vi "Read Calibration Routine.vi"(8 "error in":errorcluster, 11 "Calibration Actor in":refnum<class "Calibration Actor.lvclass">) -> (0 "error out":errorcluster, 1 "Vals":string[](array[string]), 2 "tags":string[](array[string]), 3 "Calibration Actor out":refnum<class "Calibration Actor.lvclass">)   [LabVIEW 2018, in "Calibration.lvlib" / "Calibration Actor.lvclass"]
doc: "Parse the calibration file that is loaded and load the steps as necessary."
uses:
  Calibration Actor.lvclass
  <vilib>/regexp/Match Regular Expression.xnode
  Common/Wait/Wait STEP.lvclass
  Common/O2 Valve/O2 Valve STEP.lvclass
  reusable/Sequence/STEPS/STEP.lvclass
  Common/O2 Flow Rate/O2 Flow Rate STEP.lvclass
  Common/Speaker/Speaker STEP.lvclass
  Common/Filter/Filter Step/Filter STEP.lvclass
  Common/O3 Level/O3 Lamp Frequency STEP.lvclass
  Common/O3 Generator Power/O3 Generator Power STEP.lvclass
  reusable/Sequence/SEQ/SEQ.lvclass
  <vilib>/ActorFramework/Actor/Actor.lvclass
  Common/Set cycle state/Set cycle state STEP.lvclass
  Common/Denuder/Denuder STEP.lvclass
  reusable/Session APIs/CVT/CVT.lvclass
  Common/Reset Cycle State STEP/Reset cycle state STEP.lvclass
  Common/O3 Dump Rate Step/O3 Dump Rate STEP/O3 DumpRate STEP.lvclass
  Common/Pressure Control Rate STEP/Pressure Control Rate STEP.lvclass
  Common/Inlet STEP/Inlet STEP.lvclass
  <vilib>/ActorFramework/Message Enqueuer/Message Enqueuer.lvclass
  C:/Users/Labview/Documents/exscalabar_server/reusable/Sequence/STEPS/LEAVES/Switch/Switch Step.lvclass
  C:/Users/Labview/Documents/exscalabar_server/reusable/Sequence/STEPS/STEP.lvclass
  C:/Users/Labview/Documents/exscalabar_server/reusable/Sequence/STEPS/LEAVES/Double/Switch DBL.lvclass
  C:/Users/Labview/Documents/exscalabar_server/SuperActor/SuperActor.lvclass
  C:/Program Files (x86)/National Instruments/LabVIEW 2018/vi.lib/ActorFramework/Actor/Actor.lvclass
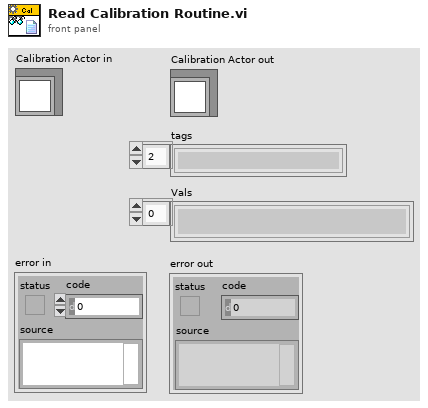
[diagram p1: front panel]
types:
  T1 = cluster{"Cycle":bool, "Period":i16, "Length":i16}
  T2 = typedef "Session - Root.lvclass/Session Handle.ctl" = refnum<data-value>
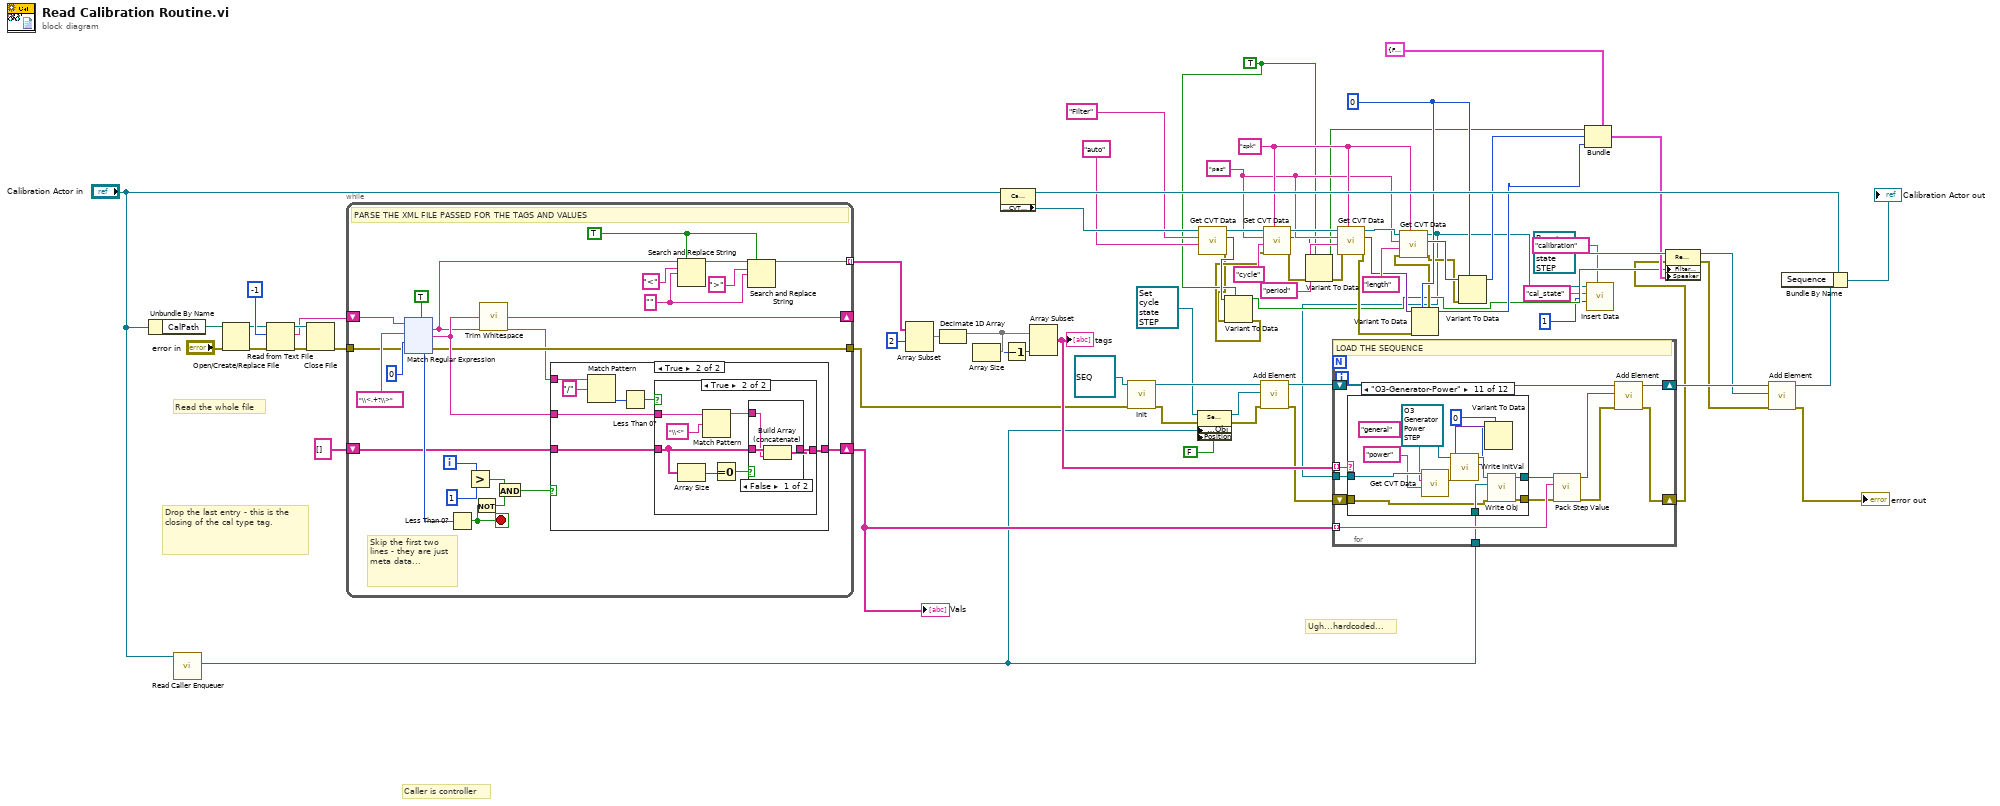
[diagram p0: block diagram]
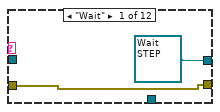
[diagram p2: hidden frame]
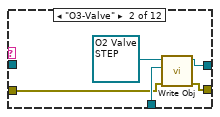
[diagram p3: hidden frame]
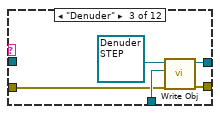
[diagram p4: hidden frame]
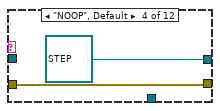
[diagram p5: hidden frame]
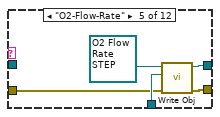
[diagram p6: hidden frame]
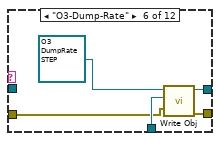
[diagram p7: hidden frame]
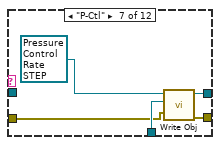
[diagram p8: hidden frame]
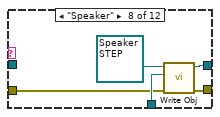
[diagram p9: hidden frame]
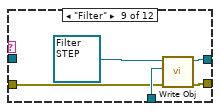
[diagram p10: hidden frame]
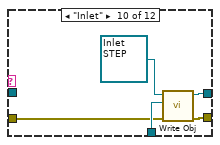
[diagram p11: hidden frame]
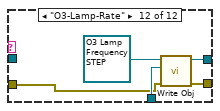
[diagram p12: hidden frame]
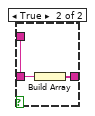
[diagram p15: hidden frame]
diagram:
  w22 = i16 0
  w27 = TRUE
  w33 = "pas" ("Group")
  w34 = "spk" ("Subgroup")
  # "Caller is controller"
  # "Ugh...hardcoded..."
  # "Read the whole file"
  # "Drop the last entry - this is the closing of the cal type tag."
  n1 = Unbundle By Name("Calibration Actor in") -> ("CalPath"=w44:path)
  n2 = call <vilib>:"Read Caller Enqueuer.vi"("Actor"="Calibration Actor in") -> ("Caller Enqueuer"=w50:refnum<class "Message Enqueuer.lvclass">)  [unwired: 10 in]
  n3 = Open/Create/Replace File(file path (use dialog)=w44, error in="error in") -> (refnum out=w71:refnum<file>, error out=w70:errorcluster)  [unwired: 4 in, 1 out]
  n4 = Read from Text File(file (use dialog)=w71, count=-1, error in=w70) -> (refnum out=w69:refnum<file>, text=w68:string, error out=w61:errorcluster)  [unwired: 1 in, 1 out]
  n5 = Close File(refnum=w69, error in=w61) -> (error out=w60:errorcluster)  [unwired: 1 out]
  n6 = while {
    shift-right: [w96] -> _
    shift-left: w68 -> [w95]
    shift-right: [w85] -> w55
    shift-left: string[] [] -> [w86]
    tunnel: w60 -> [w82]
    tunnel: [w81] -> w48
    tunnel: [w77] -> w59 mode=indexing
    i -> [w90]
    stop <- w83 stop-if-true
    w74 = "" ("replace string (\"\")")
    w76 = TRUE ("ignore case? (F)")
    # "Skip the first two lines - they are just meta data..."
    # "PARSE THE XML FILE PASSED FOR THE TAGS AND VALUES"
    n7 = xnode "Match Regular Expression"("input string"=w95, "regular expression"="\\<.+?\\>", "offset (0)"=0, "error in"=w82, "multiline? (F)"=TRUE) -> ("whole match"=w80:string, "after match"=w92:string, "offset past match"=w93:i32, "error out"=w81:errorcluster)  [unwired: 1 in, 1 out]
    n8 = Less Than 0?(x=w93) -> (x < 0?=w83:bool)
    n9 = Greater?(x=w90, y=1) -> (0:w88:bool)
    n10 = Not(x=w83) -> (.not. x?=w84:bool)
    n11 = call <vilib>:"Trim Whitespace.vi"("string"=w92) -> ("trimmed string"=w96:string)  [unwired: 1 in]
    n12 = And(x=w88, y=w84) -> (x .and. y?=w87:bool)
    n13 = case shown="True" w87 {
      tunnel: w80 -> [_ w105]
      tunnel: w92 -> [_ w101]
      tunnel: w86 -> [w98 w100]
      tunnel: [w98 w99] -> w85
      frame False {
      }
      frame True {
        n14 = Match Pattern(string=w105, regular expression="/") -> (offset past match=w103:i32)  [unwired: 1 in, 3 out]
        n15 = Less Than 0?(x=w103) -> (x < 0?=w102:bool)
        n16 = case shown="True" w102 {
          tunnel: w101 -> [_ w113]
          tunnel: w100 -> [w106 w108]
          tunnel: [w106 w109] -> w99
          frame False {
          }
          frame True {
            n17 = Array Size(array=w108) -> (size(s)=w110:i32)
            n18 = Match Pattern(string=w113, regular expression="\\<") -> (before substring=w107:string)  [unwired: 1 in, 3 out]
            n19 = Equal To 0?(x=w110) -> (x = 0?=w111:bool)
            n20 = case shown="False" w111 {
              tunnel: w107 -> [w114 w118]
              tunnel: [w115 w117] -> w109
              tunnel: w108 -> [w116 _]
              frame False {
                n21 = Build Array (concatenate)(w116, w114) -> (w115:string[])
              }
              frame True {
                n22 = Build Array(w118) -> (w117:string[])
              }
            }
          }
        }
      }
    }
    n23 = Search and Replace String(replace all?=w76, input string=w80, search string="<", replace string=w74) -> (result string=w78:string)  [unwired: 4 in, 3 out]
    n24 = Search and Replace String(replace all?=w76, input string=w78, search string=">", replace string=w74) -> (result string=w77:string)  [unwired: 4 in, 3 out]
  }
  "Vals" <- w55
  n25 = Array Subset(array=w59, index=2) -> (w65:string[])  [unwired: 1 in]
  n26 = Decimate 1D Array(w65) -> (w64:string[])  [unwired: 1 out]
  n27 = Array Size(array=w64) -> (size(s)=w63:i32)
  n28 = property class="Calibration Actor"(reference="Calibration Actor in") -> (reference out=w42:refnum<class "Calibration Actor.lvclass">, "Accessors:CVT Session"=w41:T2)  [unwired: 1 in, 1 out]
  n29 = Decrement(x=w63) -> (x-1=w62:i32)
  n30 = Array Subset(array=w64, length=w62) -> (w58:string[])  [unwired: 1 in]
  "tags" <- w58
  n31 = call-dynamic "Init.vi"("error in"=w48, "SEQ in"=refnum<class "SEQ.lvclass"> refnum ("Sequence Composition:SEQ")) -> ("error out"=w47:errorcluster, "SEQ out"=w54:refnum<class "SEQ.lvclass">)  [unwired: 8 in]
  n32 = property class="Set cycle state STEP.lvclass"(reference=refnum<class "Set cycle state STEP.lvclass"> refnum ("Set cycle state STEP.lvclass"), error in=w47, "Accessors:Obj"=w50, "Position"=FALSE) -> (reference out=w49:refnum<class "Set cycle state STEP.lvclass">, error out=w46:errorcluster)
  n33 = call "Get CVT Data.vi"("Variable"="auto" ("tag"), "Group"="Filter", "CVT Session In"=w41) -> ("error out"=w25:errorcluster, "Data Out"=w28:variant, "CVT Session Out"=w40:T2)  [unwired: 5 in, 1 out]
  n34 = Variant To Data(error in=w25, type=w27, Variant=w28) -> (data=w8:bool, error out=w26:errorcluster)
  n35 = call "Add Element.vi"("error in"=w46, "STEP"=w49, "SEQ in"=w54) -> ("error out"=w45:errorcluster, "SEQ out"=w53:refnum<class "SEQ.lvclass">)  [unwired: 7 in]
  n36 = call "Get CVT Data.vi"("Subgroup"=w34, "error in"=w26, "Variable"="cycle", "Group"=w33, "CVT Session In"=w40) -> ("error out"=w30:errorcluster, "Data Out"=w29:variant, "CVT Session Out"=w36:T2)  [unwired: 3 in, 1 out]
  n37 = Variant To Data(error in=w30, type=w27, Variant=w29) -> (data=w13:bool, error out=w21:errorcluster)
  n38 = call "Get CVT Data.vi"("Subgroup"=w34, "error in"=w21, "Variable"="period", "Group"=w33, "CVT Session In"=w36) -> ("error out"=w20:errorcluster, "Data Out"=w24:variant, "CVT Session Out"=w35:T2)  [unwired: 3 in, 1 out]
  n39 = Variant To Data(error in=w20, type=w22, Variant=w24) -> (data=w9:i16, error out=w19:errorcluster)
  n40 = call "Get CVT Data.vi"("Subgroup"=w34, "error in"=w19, "Variable"="length", "Group"=w33, "CVT Session In"=w35) -> ("error out"=w18:errorcluster, "Data Out"=w23:variant, "CVT Session Out"=w4:T2)  [unwired: 3 in, 1 out]
  n41 = for {
    tunnel: w58 -> [w244] mode=indexing
    tunnel: w55 -> [w242] mode=indexing
    tunnel: w50 -> [w236]
    shift-right: [w239] -> w7
    shift-left: w45 -> [w235]
    shift-right: [w240] -> w17
    shift-left: w53 -> [w241]
    tunnel: w4 -> [w233]
    # "LOAD THE SEQUENCE"
    n42 = case shown="\"O3-Generator-Power\"" w244 {
      tunnel: [refnum<class "Wait STEP.lvclass"> refnum ("Wait") w249 w255 refnum<class "STEP.lvclass"> refnum ("Sequence Composition:STEP.lvclass") w261 w267 w272 w276 w281 w287 w299 w304] -> w243
      tunnel: w236 -> [_ w250 w256 _ w263 w268 w273 w277 w283 w288 w300 w303]
      tunnel: w235 -> [w245 w248 w253 w257 w260 w265 w270 w274 w280 w286 w297 w301]
      tunnel: [w245 w247 w252 w257 w259 w266 w271 w275 w279 w285 w298 w302] -> w234
      tunnel: w233 -> [_ _ _ _ _ _ _ _ _ _ w294 _]
      frame "Wait" {
      }
      frame "O3-Valve" {
        n43 = call "Write Obj.vi"("error in (no error)"=w248, "Obj"=w250, "STEP in"=refnum<class "O2 Valve STEP.lvclass"> refnum ("O2 Valve")) -> ("error out"=w247:errorcluster, "STEP out"=w249:refnum<class "O2 Valve STEP.lvclass">)  [unwired: 7 in]
      }
      frame "Denuder" {
        n44 = call "Write Obj.vi"("error in (no error)"=w253, "Obj"=w256, "STEP in"=refnum<class "Denuder STEP.lvclass"> refnum ("O2 Valve")) -> ("error out"=w252:errorcluster, "STEP out"=w255:refnum<class "Denuder STEP.lvclass">)  [unwired: 7 in]
      }
      frame "NOOP", Default {
      }
      frame "O2-Flow-Rate" {
        n45 = call "Write Obj.vi"("error in (no error)"=w260, "Obj"=w263, "STEP in"=refnum<class "O2 Flow Rate STEP.lvclass"> refnum ("O2 Flow Rate")) -> ("error out"=w259:errorcluster, "STEP out"=w261:refnum<class "O2 Flow Rate STEP.lvclass">)  [unwired: 7 in]
      }
      frame "O3-Dump-Rate" {
        n46 = call "Write Obj.vi"("error in (no error)"=w265, "Obj"=w268, "STEP in"=refnum<class "O3 DumpRate STEP.lvclass"> refnum ("O2 Flow Rate")) -> ("error out"=w266:errorcluster, "STEP out"=w267:refnum<class "O3 DumpRate STEP.lvclass">)  [unwired: 7 in]
      }
      frame "P-Ctl" {
        n47 = call "Write Obj.vi"("error in (no error)"=w270, "Obj"=w273, "STEP in"=refnum<class "Pressure Control Rate STEP.lvclass"> refnum ("O2 Flow Rate")) -> ("error out"=w271:errorcluster, "STEP out"=w272:refnum<class "Pressure Control Rate STEP.lvclass">)  [unwired: 7 in]
      }
      frame "Speaker" {
        n48 = call "Write Obj.vi"("error in (no error)"=w274, "Obj"=w277, "STEP in"=refnum<class "Speaker STEP.lvclass"> refnum ("Speaker")) -> ("error out"=w275:errorcluster, "STEP out"=w276:refnum<class "Speaker STEP.lvclass">)  [unwired: 7 in]
      }
      frame "Filter" {
        n49 = call "Write Obj.vi"("error in (no error)"=w280, "Obj"=w283, "STEP in"=refnum<class "Filter STEP.lvclass"> refnum ("Filter")) -> ("error out"=w279:errorcluster, "STEP out"=w281:refnum<class "Filter STEP.lvclass">)  [unwired: 7 in]
      }
      frame "Inlet" {
        n50 = call "Write Obj.vi"("error in (no error)"=w286, "Obj"=w288, "STEP in"=refnum<class "Inlet STEP.lvclass"> refnum ("Filter")) -> ("error out"=w285:errorcluster, "STEP out"=w287:refnum<class "Inlet STEP.lvclass">)  [unwired: 7 in]
      }
      frame "O3-Generator-Power" {
        n51 = call "Get CVT Data.vi"("Variable"="power" ("tag"), "Group"="general", "CVT Session In"=w294) -> ("Data Out"=w291:variant)  [unwired: 5 in, 3 out]
        n52 = Variant To Data(type=u8 0, Variant=w291) -> (data=w289:u8)  [unwired: 1 in, 1 out]
        n53 = call-dynamic "Write InitVal.vi"("InitVal"=w289, "O3 Generator Power STEP in"=refnum<class "O3 Generator Power STEP.lvclass"> refnum ("O3 Generator Power")) -> ("O3 Generator Power STEP out"=w295:refnum<class "O3 Generator Power STEP.lvclass">)  [unwired: 8 in, 1 out]
        n54 = call "Write Obj.vi"("error in (no error)"=w297, "Obj"=w300, "STEP in"=w295) -> ("error out"=w298:errorcluster, "STEP out"=w299:refnum<class "O3 Generator Power STEP.lvclass">)  [unwired: 7 in]
      }
      frame "O3-Lamp-Rate" {
        n55 = call "Write Obj.vi"("error in (no error)"=w301, "Obj"=w303, "STEP in"=refnum<class "O3 Lamp Frequency STEP.lvclass"> refnum ("O3 Level")) -> ("error out"=w302:errorcluster, "STEP out"=w304:refnum<class "O3 Lamp Frequency STEP.lvclass">)  [unwired: 7 in]
      }
    }
    n56 = call-dynamic "Pack Step Value.vi"("error in (no error)"=w234, "Value"=w242, "STEP in"=w243) -> ("error out"=w237:errorcluster, "STEP out"=w238:refnum<class "STEP.lvclass">)  [unwired: 7 in]
    n57 = call "Add Element.vi"("error in"=w237, "STEP"=w238, "SEQ in"=w241) -> ("error out"=w239:errorcluster, "SEQ out"=w240:refnum<class "SEQ.lvclass">)  [unwired: 7 in]
  }
  n58 = Variant To Data(error in=w18, type=w22, Variant=w23) -> (data=w10:i16)  [unwired: 1 out]
  n59 = Bundle(cluster=T1 {"Cycle"=FALSE, "Period"=0, "Length"=0} ("Speaker"), "Cycle"=w13, "Period"=w10, "Length"=w9) -> (w11:T1)
  n60 = call "Insert Data.vi"("Group"="calibration", "Data"=u8 1, "tag"="cal_state", "CVT Session In"=w4) -> ()  [unwired: 6 in, 2 out]
  n61 = property class="Reset cycle state STEP.lvclass"(reference=refnum<class "Reset cycle state STEP.lvclass"> refnum ("Reset cycle state STEP.lvclass"), error in=w7, "Filter Cycle"=w8, "Speaker"=w11) -> (reference out=w14:refnum<class "Reset cycle state STEP.lvclass">, error out=w6:errorcluster)
  n62 = call "Add Element.vi"("error in"=w6, "STEP"=w14, "SEQ in"=w17) -> ("error out"=→"error out":errorcluster, "SEQ out"=w16:refnum<class "SEQ.lvclass">)  [unwired: 7 in]
  n63 = Bundle By Name(cluster=w42, "Sequence"=w16) -> (→"Calibration Actor out":refnum<class "Calibration Actor.lvclass">)
